vi "ini_object_save.vi"(7 "generate error if unsuppoted data type (true)":bool=TRUE, 8 "error in":errorcluster, 10 "auto ini row":T1, 11 "refnum in":T2) -> (0 "error out":errorcluster, 3 "refnum out":T2)   [LabVIEW 2013]
uses:
  <vilib>/Utility/config.llb/Config Data RefNum.ctl
  ini_parse_row.ctl
  <vilib>/Utility/config.llb/Write Key (String).vi
  <vilib>/Utility/config.llb/Write Key (Path).vi
  <vilib>/Utility/config.llb/Write Key (Boolean).vi
  <vilib>/Utility/config.llb/Write Key (I32).vi
  <vilib>/Utility/config.llb/Write Key (Double).vi
  <vilib>/Utility/config.llb/Write Key (U32).vi
  <vilib>/Utility/config.llb/NI_LVConfig.lvlib
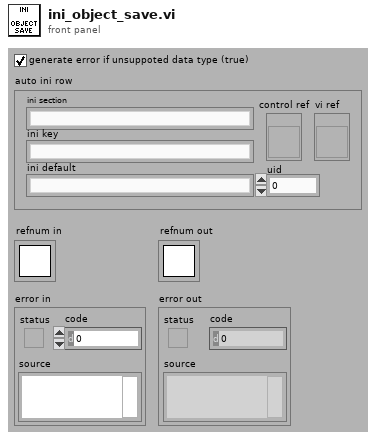
[diagram p1: front panel]
types:
  T1 = typedef "ini_parse_row.ctl" = cluster{"ini section":string, "ini key":string, "ini default":string, "control ref":refnum<vi>, "uid":i32, "vi ref":refnum<vi>}
  T2 = typedef "NI_LVConfig.lvlib/Config Data RefNum.ctl" = refnum<k1>
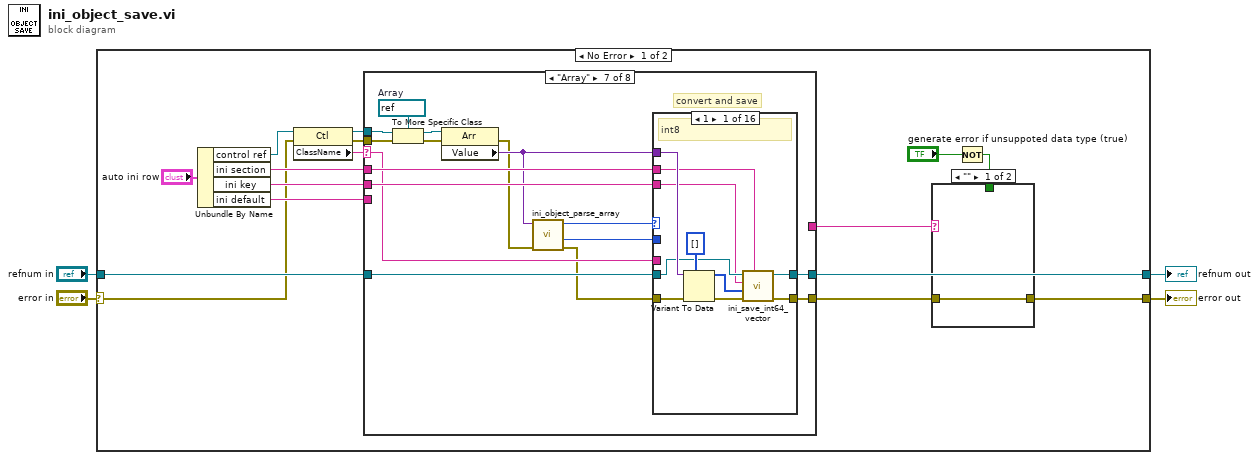
[diagram p0: block diagram]
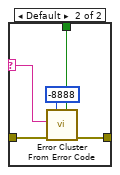
[diagram p2: hidden frame]
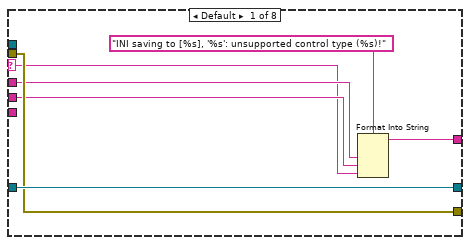
[diagram p3: hidden frame]
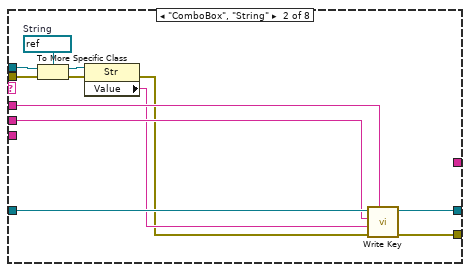
[diagram p4: hidden frame]
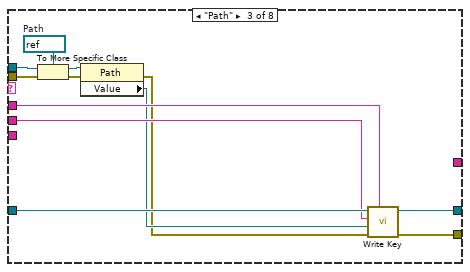
[diagram p5: hidden frame]
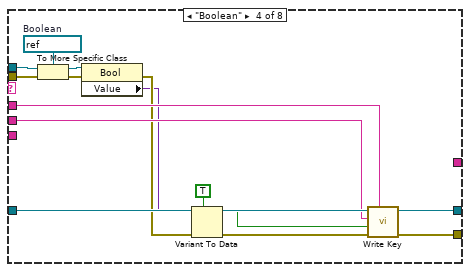
[diagram p6: hidden frame]
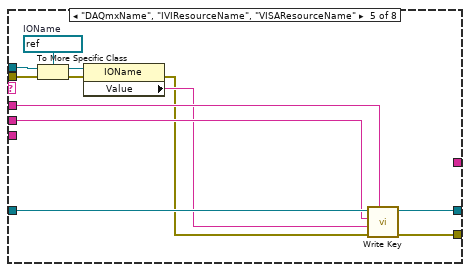
[diagram p7: hidden frame]
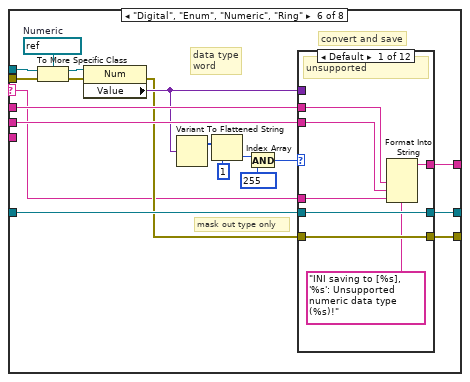
[diagram p8: hidden frame]
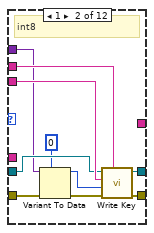
[diagram p9: hidden frame]
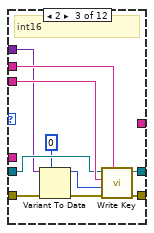
[diagram p10: hidden frame]
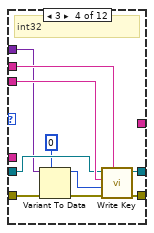
[diagram p11: hidden frame]
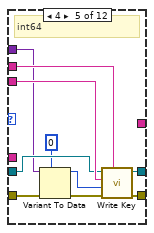
[diagram p12: hidden frame]
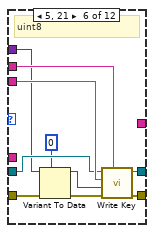
[diagram p13: hidden frame]
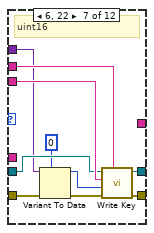
[diagram p14: hidden frame]
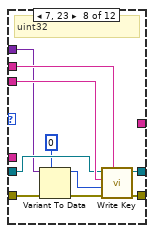
[diagram p15: hidden frame]
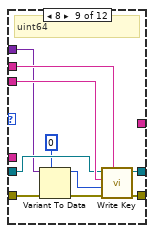
[diagram p16: hidden frame]
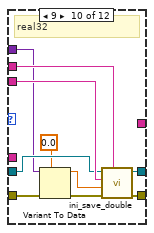
[diagram p17: hidden frame]
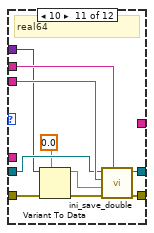
[diagram p18: hidden frame]
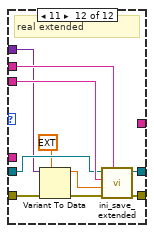
[diagram p19: hidden frame]
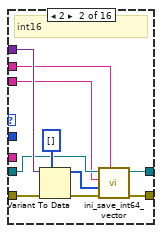
[diagram p20: hidden frame]
diagram:
  n1 = case shown="No Error" "error in" {
    selector: "error in" -> [w5 w407]
    tunnel: "refnum in" -> [w20 w406]
    tunnel: [w19 w406] -> w3
    tunnel: [w9 w407] -> w2
    frame No Error {
      n2 = Unbundle By Name("auto ini row") -> ("control ref"=w15:refnum<vi>, "ini section"=w17:string, "ini key"=w16:string, "ini default"=w13:string)
      n3 = property class="Ctl"(reference=w15, error in=w5) -> (reference out=w11:refnum<vi>, error out=w12:errorcluster, "ClassName"=w14:string)
      n4 = case shown="\"Array\"" w14 {
        selector: w14 -> [w27 _ _ _ _ w85 w226 _]
        tunnel: [w32 w45 w57 w72 w84 w103 w236 w405] -> w10
        tunnel: w20 -> [w33 w44 w56 w71 w83 w102 w235 w404]
        tunnel: [w33 w43 w55 w70 w82 w101 w234 w403] -> w19
        tunnel: w17 -> [w29 w42 w54 w69 w81 w100 w233 w402]
        tunnel: w16 -> [w28 w41 w53 w68 w80 w99 w232 w401]
        tunnel: w13 -> [_ _ _ _ _ _ _ _]
        tunnel: w12 -> [w32 w38 w50 w65 w77 w97 w230 w399]
        tunnel: w11 -> [_ w40 w52 w67 w79 w98 w231 w400]
        tunnel: [w30 _ _ _ _ w86 _ _] -> w8
        frame Default {
          n5 = Format Into String(format string="INI saving to [%s], '%s': unsupported control type (%s)!", w29, w28, w27) -> (resulting string=w30:string)  [unwired: 2 in, 1 out]
        }
        frame "ComboBox", "String" {
          w36 = refnum<vi> refnum  # String
          n6 = To More Specific Class(target class=w36, reference=w40, error in=w38) -> (specific class reference=w39:refnum<vi>, error out=w37:errorcluster)
          n7 = property class="Str"(reference=w39, error in=w37) -> (error out=w34:errorcluster, "Value"=w35:string)  [unwired: 1 out]
          n8 = call-poly <vilib>:"Write Key.vi"("section"=w42, "error in (no error)"=w34, "value"=w35, "key"=w41, "refnum"=w44) -> ("error out"=w45:errorcluster, "refnum out"=w43:T2)  [unwired: 4 in, 1 out]
        }
        frame "Path" {
          w48 = refnum<vi> refnum  # Path
          n9 = To More Specific Class(target class=w48, reference=w52, error in=w50) -> (specific class reference=w51:refnum<vi>, error out=w49:errorcluster)
          n10 = property class="Path"(reference=w51, error in=w49) -> (error out=w46:errorcluster, "Value"=w47:path)  [unwired: 1 out]
          n11 = call-poly <vilib>:"Write Key.vi"("section"=w54, "error in (no error)"=w46, "value"=w47, "key"=w53, "refnum"=w56) -> ("error out"=w57:errorcluster, "refnum out"=w55:T2)  [unwired: 4 in, 1 out]
        }
        frame "Boolean" {
          w63 = refnum<vi> refnum  # Boolean
          n12 = To More Specific Class(target class=w63, reference=w67, error in=w65) -> (specific class reference=w66:refnum<vi>, error out=w64:errorcluster)
          n13 = property class="Bool"(reference=w66, error in=w64) -> (error out=w62:errorcluster, "Value"=w59:variant)  [unwired: 1 out]
          n14 = Variant To Data(error in=w62, type=TRUE, Variant=w59) -> (data=w60:bool, error out=w61:errorcluster)
          n15 = call-poly <vilib>:"Write Key.vi"("section"=w69, "error in (no error)"=w61, "value"=w60, "key"=w68, "refnum"=w71) -> ("error out"=w72:errorcluster, "refnum out"=w70:T2)  [unwired: 4 in, 1 out]
        }
        frame "DAQmxName", "IVIResourceName", "VISAResourceName" {
          w75 = refnum<vi> refnum  # IOName
          n16 = To More Specific Class(target class=w75, reference=w79, error in=w77) -> (specific class reference=w78:refnum<vi>, error out=w76:errorcluster)
          n17 = property class="IOName"(reference=w78, error in=w76) -> (error out=w73:errorcluster, "Value"=w74:string)  [unwired: 1 out]
          n18 = call-poly <vilib>:"Write Key.vi"("section"=w81, "error in (no error)"=w73, "value"=w74, "key"=w80, "refnum"=w83) -> ("error out"=w84:errorcluster, "refnum out"=w82:T2)  [unwired: 4 in, 1 out]
        }
        frame "Digital", "Enum", "Numeric", "Ring" {
          w96 = refnum<vi> refnum  # Numeric
          # "convert and save"
          # "data type\nword"
          # "mask out type only"
          n19 = To More Specific Class(target class=w96, reference=w98, error in=w97) -> (specific class reference=w94:refnum<vi>, error out=w95:errorcluster)
          n20 = property class="Num"(reference=w94, error in=w95) -> (error out=w87:errorcluster, "Value"=w88:variant)  [unwired: 1 out]
          n21 = Variant To Flattened String(Variant=w88) -> (1:w93:i16[])  [unwired: 1 out]
          n22 = Index Array(array=w93, index=1) -> (element=w91:i16)
          n23 = And(x=w91, y=i16 255) -> (x .and. y?=w90:i16)
          n24 = case shown="Default" w90 {
            tunnel: w87 -> [w109 w116 w126 w136 w146 w156 w166 w176 w186 w196 w206 w216]
            tunnel: [w109 w120 w130 w140 w150 w160 w170 w180 w190 w200 w210 w220] -> w103
            tunnel: w102 -> [w110 w113 w123 w133 w143 w153 w163 w173 w183 w194 w203 w213]
            tunnel: [w110 w119 w129 w139 w149 w159 w169 w179 w189 w199 w209 w219] -> w101
            tunnel: w100 -> [w106 w118 w128 w138 w148 w158 w168 w178 w188 w198 w208 w218]
            tunnel: w99 -> [w105 w117 w127 w137 w147 w157 w167 w177 w187 w197 w207 w217]
            tunnel: w88 -> [_ w112 w122 w132 w142 w152 w162 w172 w182 w193 w202 w212]
            tunnel: [w108 _ _ _ _ _ _ _ _ _ _ _] -> w86
            tunnel: w85 -> [w104 _ _ _ _ _ _ _ _ _ _ _]
            frame Default {
              # "unsupported"
              n25 = Format Into String(format string="INI saving to [%s], '%s': Unsupported numeric data type (%s)!", w106, w105, w104) -> (resulting string=w108:string)  [unwired: 2 in, 1 out]
            }
            frame 1 {
              # "int8"
              n26 = Variant To Data(error in=w116, type=i8 0, Variant=w112) -> (data=w114:i8, error out=w115:errorcluster)
              n27 = call-poly <vilib>:"Write Key.vi"("section"=w118, "error in (no error)"=w115, "value"=w114, "key"=w117, "refnum"=w113) -> ("error out"=w120:errorcluster, "refnum out"=w119:T2)  [unwired: 4 in, 1 out]
            }
            frame 2 {
              # "int16"
              n28 = Variant To Data(error in=w126, type=i16 0, Variant=w122) -> (data=w124:i16, error out=w125:errorcluster)
              n29 = call-poly <vilib>:"Write Key.vi"("section"=w128, "error in (no error)"=w125, "value"=w124, "key"=w127, "refnum"=w123) -> ("error out"=w130:errorcluster, "refnum out"=w129:T2)  [unwired: 4 in, 1 out]
            }
            frame 3 {
              # "int32"
              n30 = Variant To Data(error in=w136, type=0, Variant=w132) -> (data=w134:i32, error out=w135:errorcluster)
              n31 = call-poly <vilib>:"Write Key.vi"("section"=w138, "error in (no error)"=w135, "value"=w134, "key"=w137, "refnum"=w133) -> ("error out"=w140:errorcluster, "refnum out"=w139:T2)  [unwired: 4 in, 1 out]
            }
            frame 4 {
              # "int64"
              n32 = Variant To Data(error in=w146, type=i64 0, Variant=w142) -> (data=w144:i64, error out=w145:errorcluster)
              n33 = call-poly <vilib>:"Write Key.vi"("section"=w148, "error in (no error)"=w145, "value"=w144, "key"=w147, "refnum"=w143) -> ("error out"=w150:errorcluster, "refnum out"=w149:T2)  [unwired: 4 in, 1 out]
            }
            frame 5, 21 {
              # "uint8"
              n34 = Variant To Data(error in=w156, type=u8 0, Variant=w152) -> (data=w154:u8, error out=w155:errorcluster)
              n35 = call-poly <vilib>:"Write Key.vi"("section"=w158, "error in (no error)"=w155, "value"=w154, "key"=w157, "refnum"=w153) -> ("error out"=w160:errorcluster, "refnum out"=w159:T2)  [unwired: 4 in, 1 out]
            }
            frame 6, 22 {
              # "uint16"
              n36 = Variant To Data(error in=w166, type=u16 0, Variant=w162) -> (data=w164:u16, error out=w165:errorcluster)
              n37 = call-poly <vilib>:"Write Key.vi"("section"=w168, "error in (no error)"=w165, "value"=w164, "key"=w167, "refnum"=w163) -> ("error out"=w170:errorcluster, "refnum out"=w169:T2)  [unwired: 4 in, 1 out]
            }
            frame 7, 23 {
              # "uint32"
              n38 = Variant To Data(error in=w176, type=u32 0, Variant=w172) -> (data=w174:u32, error out=w175:errorcluster)
              n39 = call-poly <vilib>:"Write Key.vi"("section"=w178, "error in (no error)"=w175, "value"=w174, "key"=w177, "refnum"=w173) -> ("error out"=w180:errorcluster, "refnum out"=w179:T2)  [unwired: 4 in, 1 out]
            }
            frame 8 {
              # "uint64"
              n40 = Variant To Data(error in=w186, type=u64 0, Variant=w182) -> (data=w184:u64, error out=w185:errorcluster)
              n41 = call-poly <vilib>:"Write Key.vi"("section"=w188, "error in (no error)"=w185, "value"=w184, "key"=w187, "refnum"=w183) -> ("error out"=w190:errorcluster, "refnum out"=w189:T2)  [unwired: 4 in, 1 out]
            }
            frame 9 {
              # "real32"
              n42 = Variant To Data(error in=w196, type=sgl 0.0, Variant=w193) -> (data=w191:sgl, error out=w195:errorcluster)
              n43 = call "ini_save_double.vi"("section"=w198, "error in"=w195, "double"=w191, "key"=w197, "refnum in"=w194) -> ("error out"=w200:errorcluster, "refnum out"=w199:T2)  [unwired: 4 in, 1 out]
            }
            frame 10 {
              # "real64"
              n44 = Variant To Data(error in=w206, type=0.0, Variant=w202) -> (data=w204:dbl, error out=w205:errorcluster)
              n45 = call "ini_save_double.vi"("section"=w208, "error in"=w205, "double"=w204, "key"=w207, "refnum in"=w203) -> ("error out"=w210:errorcluster, "refnum out"=w209:T2)  [unwired: 4 in, 1 out]
            }
            frame 11 {
              # "real extended"
              n46 = Variant To Data(error in=w216, type=ext 0.0, Variant=w212) -> (data=w214:ext, error out=w215:errorcluster)
              n47 = call "ini_save_extended.vi"("section"=w218, "error in"=w215, "double"=w214, "key"=w217, "refnum in"=w213) -> ("error out"=w220:errorcluster, "refnum out"=w219:T2)  [unwired: 4 in, 1 out]
            }
          }
        }
        frame "Array" {
          w229 = refnum<vi> refnum  # Array
          # "convert and save"
          n48 = To More Specific Class(target class=w229, reference=w231, error in=w230) -> (specific class reference=w227:refnum<vi>, error out=w228:errorcluster)
          n49 = property class="Arr"(reference=w227, error in=w228) -> (error out=w223:errorcluster, "Value"=w225:variant)  [unwired: 1 out]
          n50 = call "ini_object_parse_array.vi"("error in"=w223, "variant in"=w225) -> ("error out"=w222:errorcluster, "dims"=w221:i16, "type id"=w224:i16)  [unwired: 6 in, 1 out]
          n51 = case shown="1" w224 {
            tunnel: w222 -> [w246 w256 w266 w276 w282 w292 w302 w312 w322 w332 w342 w352 w362 w372 w382 w393]
            tunnel: [w243 w253 w263 w273 w286 w296 w306 w316 w326 w336 w346 w356 w366 w376 w386 w392] -> w236
            tunnel: w235 -> [w239 w249 w259 w269 w280 w290 w299 w309 w319 w329 w339 w349 w359 w369 w380 w390]
            tunnel: [w242 w252 w262 w272 w285 w295 w305 w315 w325 w335 w345 w355 w365 w375 w385 w391] -> w234
            tunnel: w233 -> [w240 w250 w260 w270 w284 w294 w304 w314 w324 w334 w344 w354 w364 w374 w384 w389]
            tunnel: w232 -> [w238 w248 w258 w268 w283 w293 w303 w313 w323 w333 w343 w353 w363 w373 w383 w388]
            tunnel: w225 -> [w245 w255 w265 w275 w279 w289 w298 w308 w318 w328 w338 w348 w358 w368 w379 w387]
            tunnel: w226 -> [_ _ _ _ _ _ _ _ _ _ _ _ _ _ _ _]
            tunnel: w221 -> [_ _ _ _ _ _ _ _ _ _ _ _ _ _ _ _]
            frame 1 {
              # "int8"
              n52 = Variant To Data(error in=w246, type=i8[] [], Variant=w245) -> (data=w237:i8[], error out=w241:errorcluster)
              n53 = call "ini_save_int64_vector.vi"("section"=w240, "error in"=w241, "values"=w237, "key"=w238, "refnum in"=w239) -> ("error out"=w243:errorcluster, "refnum out"=w242:T2)  [unwired: 4 in, 1 out]
            }
            frame 2 {
              # "int16"
              n54 = Variant To Data(error in=w256, type=i16[] [], Variant=w255) -> (data=w247:i16[], error out=w251:errorcluster)
              n55 = call "ini_save_int64_vector.vi"("section"=w250, "error in"=w251, "values"=w247, "key"=w248, "refnum in"=w249) -> ("error out"=w253:errorcluster, "refnum out"=w252:T2)  [unwired: 4 in, 1 out]
            }
            frame 3 {
              # "int32"
              n56 = Variant To Data(error in=w266, type=i32[] [], Variant=w265) -> (data=w257:i32[], error out=w261:errorcluster)
              n57 = call "ini_save_int64_vector.vi"("section"=w260, "error in"=w261, "values"=w257, "key"=w258, "refnum in"=w259) -> ("error out"=w263:errorcluster, "refnum out"=w262:T2)  [unwired: 4 in, 1 out]
            }
            frame 4 {
              # "int64"
              n58 = Variant To Data(error in=w276, type=i64[] [], Variant=w275) -> (data=w267:i64[], error out=w271:errorcluster)
              n59 = call "ini_save_int64_vector.vi"("section"=w270, "error in"=w271, "values"=w267, "key"=w268, "refnum in"=w269) -> ("error out"=w273:errorcluster, "refnum out"=w272:T2)  [unwired: 4 in, 1 out]
            }
            frame 5, 21 {
              # "uint8"
              n60 = Variant To Data(error in=w282, type=u8[] [], Variant=w279) -> (data=w277:u8[], error out=w281:errorcluster)
              n61 = call "ini_save_uint64_vector.vi"("section"=w284, "error in"=w281, "values"=w277, "key"=w283, "refnum in"=w280) -> ("error out"=w286:errorcluster, "refnum out"=w285:T2)  [unwired: 4 in, 1 out]
            }
            frame 6, 22 {
              # "uint16"
              n62 = Variant To Data(error in=w292, type=u16[] [], Variant=w289) -> (data=w287:u16[], error out=w291:errorcluster)
              n63 = call "ini_save_uint64_vector.vi"("section"=w294, "error in"=w291, "values"=w287, "key"=w293, "refnum in"=w290) -> ("error out"=w296:errorcluster, "refnum out"=w295:T2)  [unwired: 4 in, 1 out]
            }
            frame 7, 23 {
              # "uint32"
              n64 = Variant To Data(error in=w302, type=u32[] [], Variant=w298) -> (data=w300:u32[], error out=w301:errorcluster)
              n65 = call "ini_save_uint64_vector.vi"("section"=w304, "error in"=w301, "values"=w300, "key"=w303, "refnum in"=w299) -> ("error out"=w306:errorcluster, "refnum out"=w305:T2)  [unwired: 4 in, 1 out]
            }
            frame 8 {
              # "uint64"
              n66 = Variant To Data(error in=w312, type=u64[] [], Variant=w308) -> (data=w310:u64[], error out=w311:errorcluster)
              n67 = call "ini_save_uint64_vector.vi"("section"=w314, "error in"=w311, "values"=w310, "key"=w313, "refnum in"=w309) -> ("error out"=w316:errorcluster, "refnum out"=w315:T2)  [unwired: 4 in, 1 out]
            }
            frame 9 {
              # "real32"
              n68 = Variant To Data(error in=w322, type=sgl[] [], Variant=w318) -> (data=w320:sgl[], error out=w321:errorcluster)
              n69 = call "ini_save_double_vector.vi"("section"=w324, "error in"=w321, "values"=w320, "key"=w323, "refnum in"=w319) -> ("error out"=w326:errorcluster, "refnum out"=w325:T2)  [unwired: 4 in, 1 out]
            }
            frame 10 {
              # "real64"
              n70 = Variant To Data(error in=w332, type=dbl[] [], Variant=w328) -> (data=w330:dbl[], error out=w331:errorcluster)
              n71 = call "ini_save_double_vector.vi"("section"=w334, "error in"=w331, "values"=w330, "key"=w333, "refnum in"=w329) -> ("error out"=w336:errorcluster, "refnum out"=w335:T2)  [unwired: 4 in, 1 out]
            }
            frame 11 {
              # "real extended"
              n72 = Variant To Data(error in=w342, type=ext[] [], Variant=w338) -> (data=w340:ext[], error out=w341:errorcluster)
              n73 = call "ini_save_extended_vector.vi"("section"=w344, "error in"=w341, "values"=w340, "key"=w343, "refnum in"=w339) -> ("error out"=w346:errorcluster, "refnum out"=w345:T2)  [unwired: 4 in, 1 out]
            }
            frame 12 {
              # "cplx single"
              n74 = Variant To Data(error in=w352, type=csg[] [], Variant=w348) -> (data=w350:csg[], error out=w351:errorcluster)
              n75 = call "ini_save_cplx_double_vector.vi"("section"=w354, "error in"=w351, "values"=w350, "key"=w353, "refnum in"=w349) -> ("error out"=w356:errorcluster, "refnum out"=w355:T2)  [unwired: 4 in, 1 out]
            }
            frame 13 {
              # "cplx double"
              n76 = Variant To Data(error in=w362, type=cdb[] [], Variant=w358) -> (data=w360:cdb[], error out=w361:errorcluster)
              n77 = call "ini_save_cplx_double_vector.vi"("section"=w364, "error in"=w361, "values"=w360, "key"=w363, "refnum in"=w359) -> ("error out"=w366:errorcluster, "refnum out"=w365:T2)  [unwired: 4 in, 1 out]
            }
            frame 14 {
              # "cplx extended"
              n78 = Variant To Data(error in=w372, type=cxt[] [], Variant=w368) -> (data=w370:cxt[], error out=w371:errorcluster)
              n79 = call "ini_save_cplx_extended_vector.vi"("section"=w374, "error in"=w371, "values"=w370, "key"=w373, "refnum in"=w369) -> ("error out"=w376:errorcluster, "refnum out"=w375:T2)  [unwired: 4 in, 1 out]
            }
            frame 48, 55 {
              # "string"
              n80 = Variant To Data(error in=w382, type=string[] [], Variant=w379) -> (data=w377:string[], error out=w381:errorcluster)
              n81 = call "ini_save_string_vector.vi"("section"=w384, "error in"=w381, "values"=w377, "key"=w383, "refnum in"=w380) -> ("error out"=w386:errorcluster, "refnum out"=w385:T2)  [unwired: 4 in, 1 out]
            }
            frame Default {
              # "unknown"
              n82 = call "ini_save_variant.vi"("section"=w389, "error in"=w393, "Variant"=w387, "key"=w388, "refnum in"=w390) -> ("error out"=w392:errorcluster, "refnum out"=w391:T2)  [unwired: 4 in, 1 out]
            }
          }
        }
        frame "Cluster" {
          w398 = refnum<vi> refnum  # Cluster
          n83 = To More Specific Class(target class=w398, reference=w400, error in=w399) -> (specific class reference=w396:refnum<vi>, error out=w397:errorcluster)
          n84 = property class="Clust"(reference=w396, error in=w397) -> (error out=w394:errorcluster, "Value"=w395:variant)  [unwired: 1 out]
          n85 = call "ini_save_variant.vi"("section"=w402, "error in"=w394, "Variant"=w395, "key"=w401, "refnum in"=w404) -> ("error out"=w405:errorcluster, "refnum out"=w403:T2)  [unwired: 4 in, 1 out]
        }
      }
      n86 = Not(x="generate error if unsuppoted data type (true)") -> (.not. x?=w6:bool)
      n87 = case shown="\"\"" w8 {
        selector: w8 -> [_ w23]
        tunnel: w10 -> [w21 w26]
        tunnel: [w21 w25] -> w9
        tunnel: w6 -> [_ w22]
        frame "" {
        }
        frame Default {
          n88 = call <vilib>:"Error Cluster From Error Code.vi"("is warning? (False)"=w22, "error in (no error)"=w26, "error message (\"\")"=w23, "error code (0)"=-8888) -> ("error out"=w25:errorcluster)  [unwired: 5 in]
        }
      }
    }
    frame Error {
    }
  }
  "error out" <- w2
  "refnum out" <- w3
